vi "Move Relative (SubVI).vi"(3 "error in (no error)":errorcluster, 4 "Degrees to move":dbl, 5 "VISA resource name":refnum<visa-resource-name>) -> (0 "error out":errorcluster, 1 "New Angle":dbl, 2 "VISA resource name out":refnum<visa-resource-name>)   [LabVIEW 2012]
uses:
  <instrlib>/ZaberTSeries/Public/Utility/Request.ctl
  <instrlib>/ZaberTSeries/ZaberTSeries.lvlib
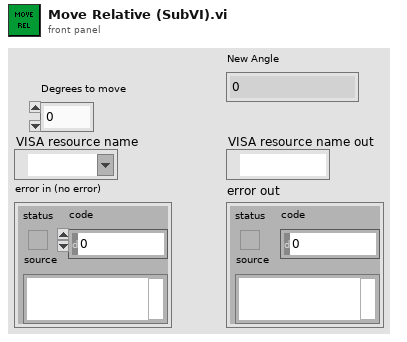
[diagram p1: front panel]
types:
  T1 = typedef "ZaberTSeries.lvlib/Request.ctl" = cluster{"Device Number":u8, "Command":u8, "Data":i32, "Response Count":i32}
  T2 = typedef "ZaberTSeries.lvlib/Response.ctl" = cluster{"Device Number":u8, "Command":u8, "Data":i32}
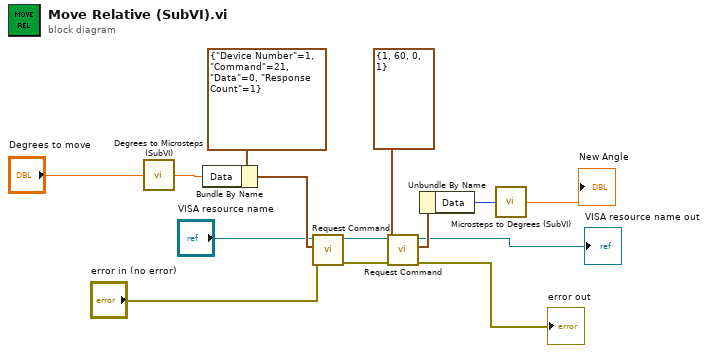
[diagram p0: block diagram]
diagram:
  n1 = call "Degrees to Microsteps (SubVI).vi"("Degrees"="Degrees to move") -> ("Microsteps"=w12:dbl)  [unwired: 4 in]
  n2 = Bundle By Name(cluster=T1 {"Device Number"=1, "Command"=21, "Data"=0, "Response Count"=1} ("Request"), "Data"=w12) -> (w11:T1)
  n3 = call <instrlib>:"Request Command.vi"("error in (no error)"="error in (no error)", "Request"=w11, "VISA resource name"="VISA resource name") -> ("error out"=w10:errorcluster, "VISA resource name out"=w9:refnum<visa-resource-name>)  [unwired: 5 in, 2 out]
  n4 = call <instrlib>:"Request Command.vi"("error in (no error)"=w10, "Request"=T1 {"Device Number"=1, "Command"=60, "Data"=0, "Response Count"=1}, "VISA resource name"=w9) -> ("error out"=→"error out":errorcluster, "First Response"=w7:T2, "VISA resource name out"=→"VISA resource name out":refnum<visa-resource-name>)  [unwired: 5 in, 1 out]
  n5 = Unbundle By Name(w7) -> ("Data"=w6:i32)
  n6 = call "Microsteps to Degrees (SubVI).vi"("Microsteps"=w6) -> ("Numeric"=→"New Angle":dbl)  [unwired: 4 in]
